vi "subHamamatsu_Deinitialization.vi"(8 "error in (no error)":errorcluster, 11 "Handle":u32) -> (0 "error out":errorcluster)   [LabVIEW 2015]
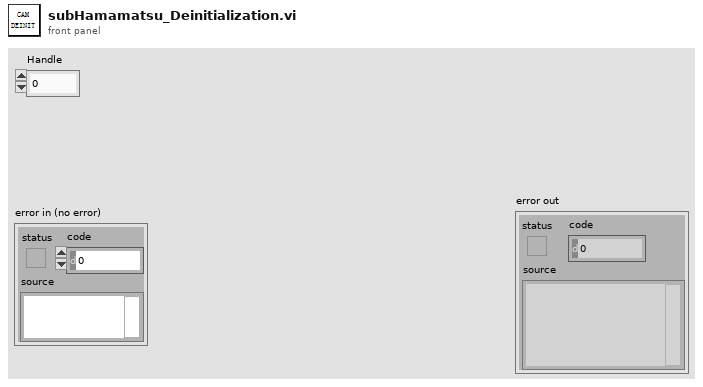
[diagram p1: front panel]
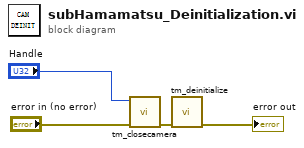
[diagram p0: block diagram]
diagram:
  n1 = call "tm_closecamera.vi"("error in (no error)"="error in (no error)", "Handle in"="Handle") -> ("error out"=w4:errorcluster)  [unwired: 9 in]
  n2 = call "tm_deinitialize.vi"("error in (no error)"=w4) -> ("error out"=→"error out":errorcluster)  [unwired: 10 in]
